vi "Scan with scanning mirror_center point_ver4.0.vi"(8 "Y Scan range (V)":dbl=0.2 min=-200.0 max=300.0, 9 "X Scan range (V)":dbl=0.2 min=-200.0 max=300.0, 10 "Y center (V)":dbl min=-200.0 max=300.0, 11 "X center (V)":dbl min=-200.0 max=300.0) -> ()   [LabVIEW 2015]
uses:
  DNV_YTW/SR400/Public/Typedefs/Counter.ctl
  <vilib>/Analysis/1siggen.llb/Ramp Pattern by Samples.vi
  <vilib>/Analysis/NI_AALBase.lvlib
  DNV_YTW/SR400/SR400.lvlib
panel:
  in  "file path":path
  out "SR400 counts":dbl
  in  "STOP\nSCAN":bool
  in  "Position from":enum16{"Left", "Right", "Control"}(ring)
  in  "Scan select":enum16{"Left", "Right"}(ring)
  in  "Position select":enum16{"Left", "Right", "Zero", "Control"}(ring)
  out "Current Y position (V)":dbl format="%#_4g"
  out "Current X position (V)":dbl format="%#_4g"
  out "Cursor_Y (V) 2":dbl format="%#.5f"
  out "Cursor_X (V) 2":dbl format="%#.5f"
  out "Cursor_Y position 2":i32
  out "Cursor_X position 2":i32
  out "X_Array 2":dbl[](array[numeric])
  out "Y_Array 2":dbl[](array[numeric])
  out "Rescanned Intensity Graph":dbl[][](graph)
  out "Count plot":dbl(graph)=137.0
  in  "stop monitoring":bool
  in  "Log":bool
  out "X_Array":dbl[](array[numeric])
  out "Y_Array":dbl[](array[numeric])
  in  "Scan":bool
  out "Cursor_Y (V)":dbl format="%#.5f"
  out "Cursor_X (V)":dbl format="%#.5f"
  in  "Go":bool
  in  "Stop program":bool
  out "Cursor_Y position":i32
  out "Cursor_X position":i32
  in  "Count Time Set":dbl[unit]=0.01
  in  "# of average":i32=1
  in  "VISA resource name":refnum<visa-resource-name>="GPIB0::23::INSTR"
  out "Counts":dbl
  in  "Time delay bet. movement\n& measurement (ms)":i32=1
  in  "X data number(Ao1)":i32=150
  out "Max Value":dbl format="%#.2p"
  out "Max Y (V)":dbl format="%#.5f"
  out "Max X (V)":dbl format="%#.5f"
  out "Intensity Graph":dbl[][](graph)
  out "ao1_V":dbl
  out "ao1_index":i32
  out "ao0_V":dbl
  out "ao0_index":i32
  in  "Y data number(Ao0)":i32=150
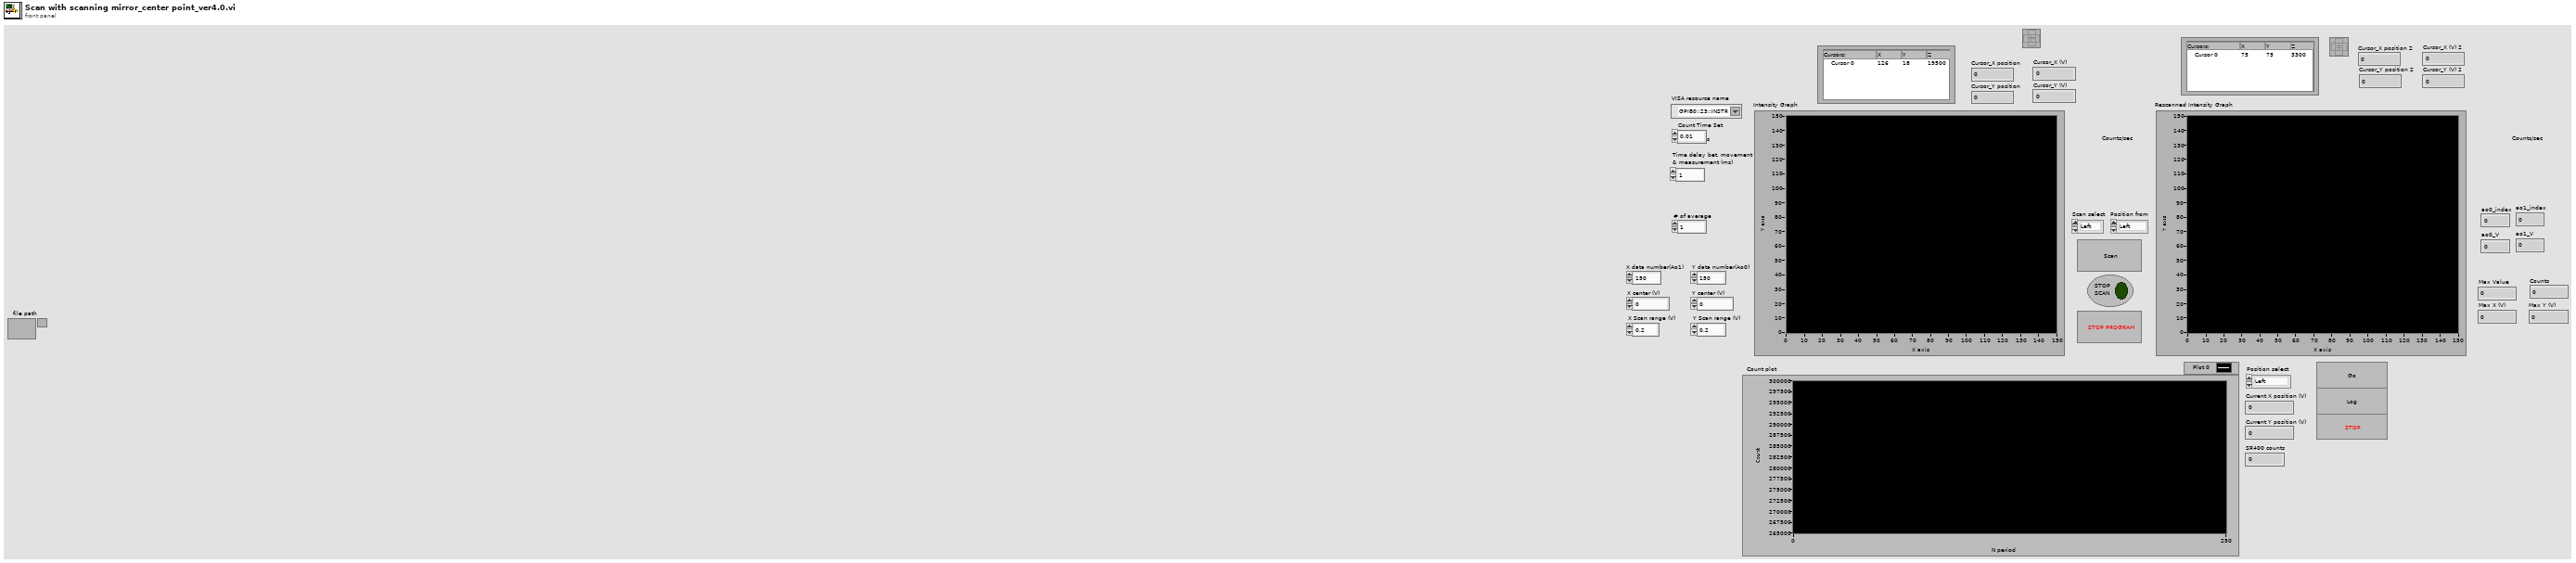
[diagram p1: front panel]
types:
  T1 = enum16{"open", "open or create", "create or replace", "create", "open (read only)"}
  T2 = typedef "SR400.lvlib/Counter.ctl" = enum16{"Counter A", "Counter B", "Counter T"}
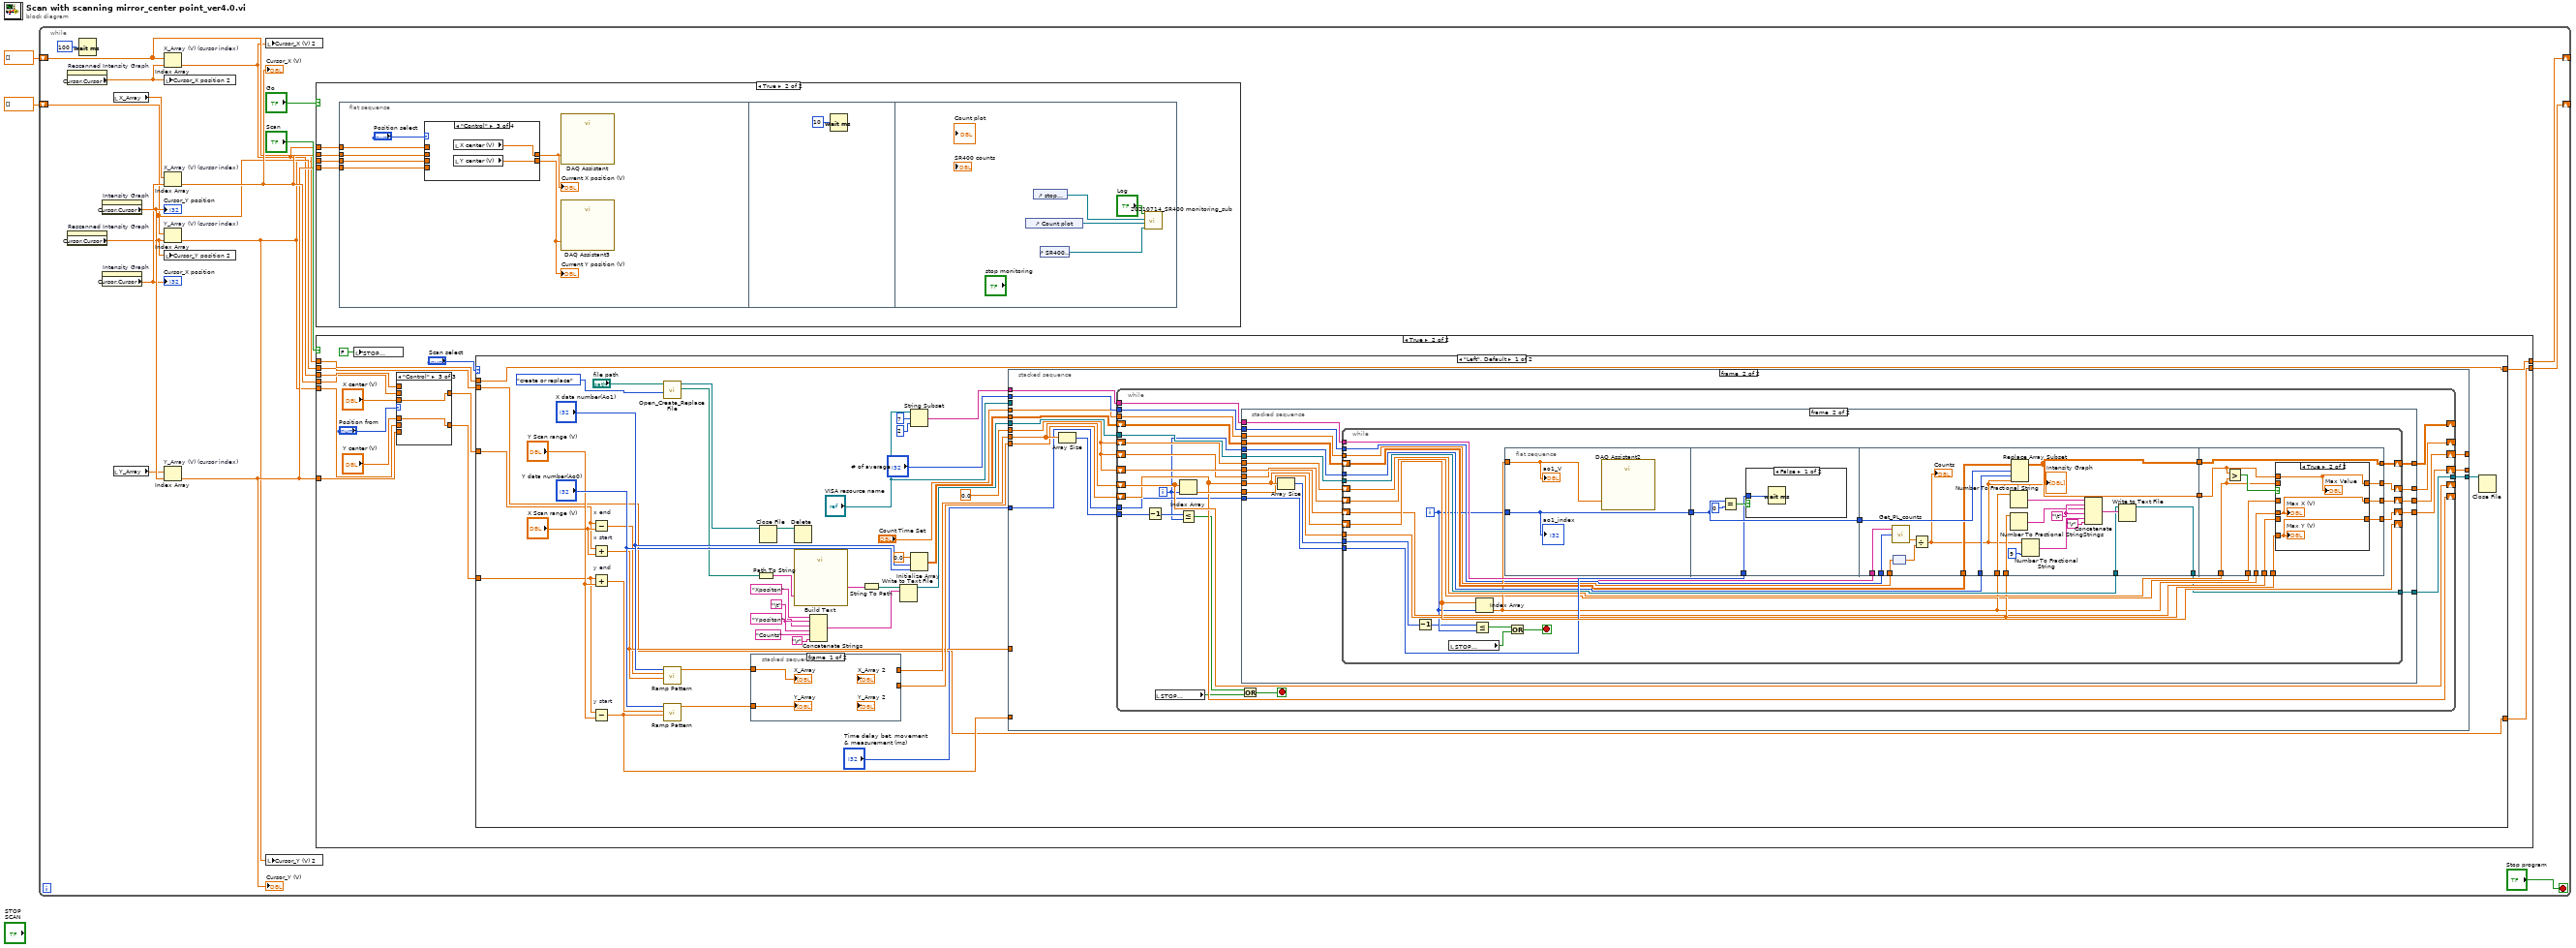
[diagram p0: block diagram]
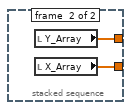
[diagram p5: hidden frame]
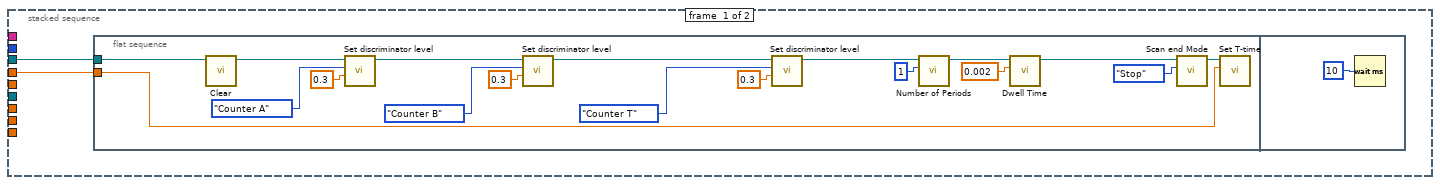
[diagram p6: hidden frame]
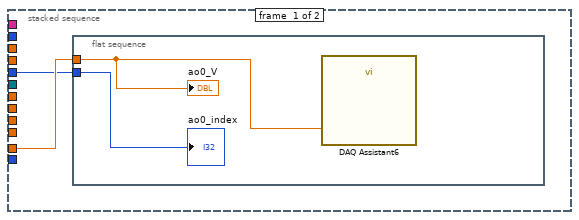
[diagram p7: hidden frame]
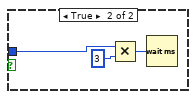
[diagram p8: hidden frame]
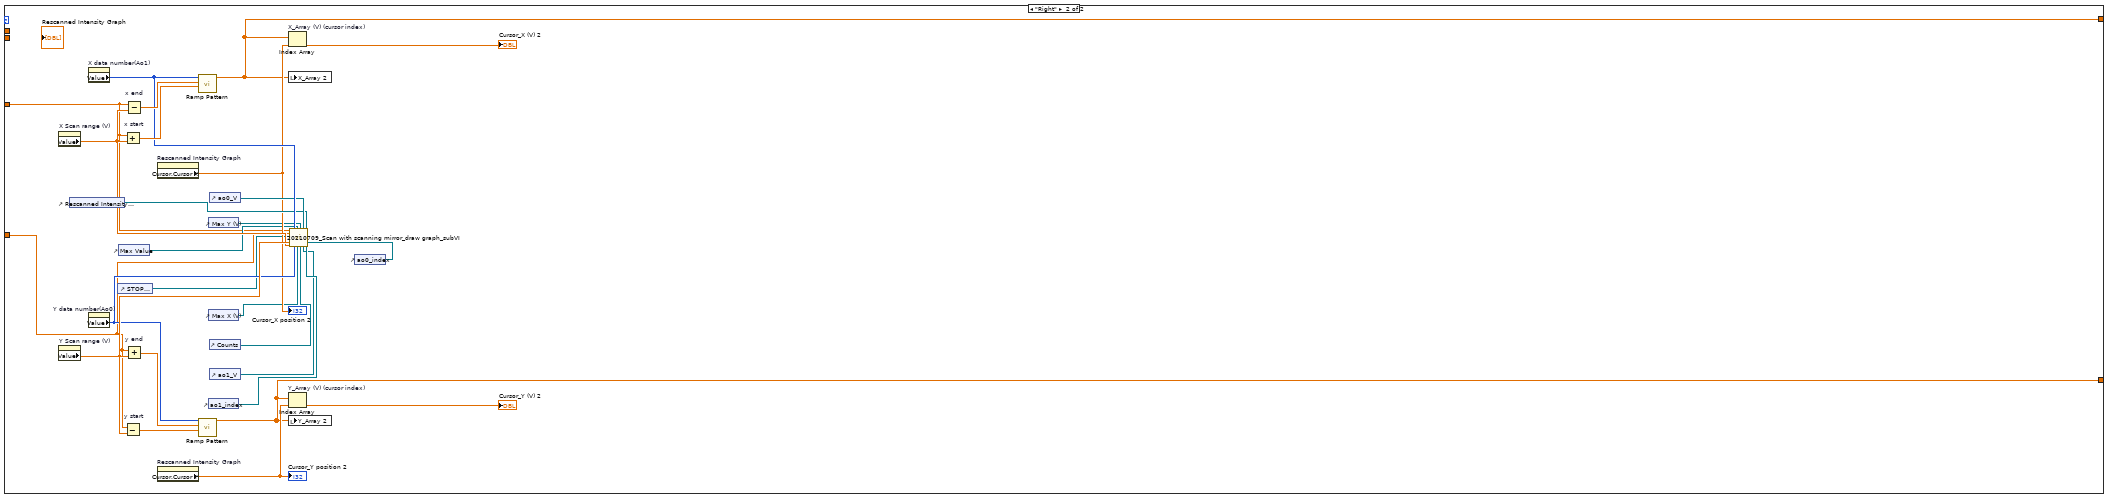
[diagram p10: hidden frame]
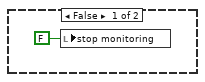
[diagram p11: hidden frame]
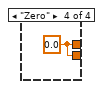
[diagram p14: hidden frame]
diagram:
  n1 = while {
    shift-right: [w10] -> _
    shift-left: dbl[] [] ("Ramp Pattern") -> [w6]
    shift-right: [w7] -> _
    shift-left: dbl[] [] ("Ramp Pattern") -> [w5]
    stop <- "Stop program" stop-if-true
    n2 = property on="Rescanned Intensity Graph" class="IntGraph (strict)"() -> ("Cursor.Cursor X"=w9:dbl)  [unwired: 2 in, 2 out]
    n3 = property on="Rescanned Intensity Graph" class="IntGraph (strict)"() -> ("Cursor.Cursor Y"=w8:dbl)  [unwired: 2 in, 2 out]
    n4 = Wait (ms)(milliseconds to wait=u32 100) -> ()  [unwired: 1 out]
    n5 = property on="Intensity Graph" class="IntGraph (strict)"() -> ("Cursor.Cursor Y"=w17:dbl)  [unwired: 2 in, 2 out]
    "Cursor_Y position" <- w17
    n6 = property on="Intensity Graph" class="IntGraph (strict)"() -> ("Cursor.Cursor X"=w16:dbl)  [unwired: 2 in, 2 out]
    "Cursor_X position" <- w16
    n7 = local read "X_Array"() -> (w15:dbl[])
    n8 = local read "Y_Array"() -> (w14:dbl[])
    n9 = Index Array "X_Array (V) (cursor index)"(array=w6, index=w9) -> (element=w4:dbl)
    n10 = local write "Cursor_X position 2"(w9) -> ()
    n11 = Index Array "X_Array (V) (cursor index)"(array=w15, index=w16) -> (element=w12:dbl)
    "Cursor_X (V)" <- w12
    n12 = Index Array "Y_Array (V) (cursor index)"(array=w5, index=w8) -> (element=w3:dbl)
    n13 = local write "Cursor_Y position 2"(w8) -> ()
    n14 = Index Array "Y_Array (V) (cursor index)"(array=w14, index=w17) -> (element=w11:dbl)
    "Cursor_Y (V)" <- w11
    n15 = local write "Cursor_X (V) 2"(w4) -> ()
    n16 = local write "Cursor_Y (V) 2"(w3) -> ()
    n17 = case shown="True" "Go" {
      tunnel: w12 -> [_ w275]
      tunnel: w11 -> [_ w274]
      tunnel: w4 -> [_ w273]
      tunnel: w3 -> [_ w272]
      frame False {
        n18 = local write "stop monitoring"(FALSE ("monitoring stop")) -> ()
      }
      frame True {
        n19 = flat-sequence {
          tunnel: w275 -> [w281]
          tunnel: w274 -> [w280]
          tunnel: w273 -> [w279]
          tunnel: w272 -> [w278]
          frame #0 {
            n20 = case shown="\"Control\"" "Position select" {
              tunnel: w281 -> [w284 _ _ _]
              tunnel: w280 -> [w283 _ _ _]
              tunnel: w279 -> [_ w286 _ _]
              tunnel: w278 -> [_ w285 _ _]
              tunnel: [w284 w286 w287 w289] -> w277
              tunnel: [w283 w285 w288 w289] -> w276
              frame "Left", Default {
              }
              frame "Right" {
              }
              frame "Control" {
                n21 = local read "X center (V)"() -> (w287:dbl)
                n22 = local read "Y center (V)"() -> (w288:dbl)
              }
              frame "Zero" {
                w289 = 0.0
              }
            }
            "Current X position (V)" <- w277
            "Current Y position (V)" <- w276
            n23 = call "DAQ Assistant"("data"=w277) -> ()  [unwired: 17 in, 2 out]
            n24 = call "DAQ Assistant3"("data"=w276) -> ()  [unwired: 17 in, 2 out]
          }
          frame #1 {
            n25 = Wait (ms)(milliseconds to wait=u32 10) -> ()  [unwired: 1 out]
          }
          frame #2 {
            n26 = control-ref of="Count plot"() -> (w294:refnum<vi>)
            n27 = control-ref of="stop monitoring"() -> (w293:refnum<vi>)
            n28 = control-ref of="SR400 counts"() -> (w291:refnum<vi>)
            n29 = call "20210714_SR400 monitoring_sub.vi"("DigNum Refnum"=w291, "Ctl Refnum"=w294, "stop Refnum"=w293, 11:"Log") -> ()  [unwired: 8 in]
          }
        }
      }
    }
    n30 = case shown="True" "Scan" {
      tunnel: w11 -> [_ w28]
      tunnel: w12 -> [_ w30]
      tunnel: [w22 w37] -> w10
      tunnel: [w21 w36] -> w7
      tunnel: w6 -> [w22 w34]
      tunnel: w5 -> [w21 w33]
      tunnel: w4 -> [_ w31]
      tunnel: w3 -> [_ w29]
      frame False {
      }
      frame True {
        n31 = local write "STOP\nSCAN"(FALSE ("STOP SCAN")) -> ()
        n32 = case shown="\"Control\"" "Position from" {
          tunnel: [w39 w41 w43] -> w27
          tunnel: w30 -> [w39 _ _]
          tunnel: w28 -> [w38 _ _]
          tunnel: [w38 w40 w42] -> w26
          tunnel: w31 -> [_ w41 _]
          tunnel: w29 -> [_ w40 _]
          tunnel: "X center (V)" -> [_ _ w43]
          tunnel: "Y center (V)" -> [_ _ w42]
          frame "Left", Default {
          }
          frame "Right" {
          }
          frame "Control" {
          }
        }
        n33 = case shown="\"Left\", Default" "Scan select" {
          tunnel: [w59 w251] -> w37
          tunnel: [w58 w250] -> w36
          tunnel: w34 -> [w59 _]
          tunnel: w33 -> [w58 _]
          tunnel: w27 -> [w53 w247]
          tunnel: w26 -> [w52 w246]
          frame "Left", Default {
            w65 = "\t"
            n34 = Subtract "x end"(x=w53, y="X Scan range (V)") -> (x-y=w72:dbl)
            n35 = Add "x start"(x=w53, y="X Scan range (V)") -> (x+y=w73:dbl)
            n36 = Add "y end"(x=w52, y="Y Scan range (V)") -> (x+y=w71:dbl)
            n37 = Subtract "y start"(x=w52, y="Y Scan range (V)") -> (x-y=w70:dbl)
            n38 = call <vilib>:"Open_Create_Replace File.vi"("function (open:0)"=T1."create or replace", "file path"="file path") -> ("new file path"=w50:path, "refnum"=w46:refnum<file>)  [unwired: 6 in, 2 out]
            n39 = call-poly <vilib>:"Ramp Pattern.vi"("start"=w73, "end"=w72, "samples"="X data number(Ao1)") -> ("Ramp Pattern"=w85:dbl[])  [unwired: 7 in, 1 out]
            n40 = call-poly <vilib>:"Ramp Pattern.vi"("start"=w70, "end"=w71, "samples"="Y data number(Ao0)") -> ("Ramp Pattern"=w84:dbl[])  [unwired: 7 in, 1 out]
            n41 = stacked-sequence {
              tunnel: [_ w89] -> w82
              tunnel: [_ w88] -> w83
              tunnel: w84 -> [w87 _]
              tunnel: w85 -> [w86 _]
              frame #0 {
                "Y_Array" <- w87
                "X_Array" <- w86
              }
              frame #1 {
                n42 = local read "Y_Array"() -> (w89:dbl[])
                n43 = local read "X_Array"() -> (w88:dbl[])
              }
            }
            n44 = Path To String(path=w50) -> (string=w45:string)
            n45 = Close File(refnum=w46) -> (path=w47:path)  [unwired: 1 in, 1 out]
            n46 = Delete(path (use dialog)=w47) -> ()  [unwired: 4 in, 3 out]
            n47 = call "Build Text"("a"=w45) -> ("Result"=w51:string)  [unwired: 13 in, 1 out]
            n48 = Concatenate Strings("Xpositon" ("string"), w65, "Ypositon" ("string"), w65, "Counts" ("string"), "\r") -> (w62:string)
            n49 = String To Path(string=w51) -> (path=w44:path)
            n50 = Write to Text File(file (use dialog)=w44, text=w62) -> (refnum out=w68:refnum<file>)  [unwired: 2 in, 2 out]
            n51 = String Subset(string="VISA resource name", offset (0)=7, length (rest)=2 ("length (rest)")) -> (substring=w55:string)
            n52 = Initialize Array(0.0, "X data number(Ao1)", "Y data number(Ao0)") -> (w77:dbl[][])
            n53 = stacked-sequence {
              tunnel: w82 -> [_ w123]
              tunnel: w83 -> [_ w122]
              tunnel: "Time delay bet. movement\n& measurement (ms)" -> [_ w121]
              tunnel: w55 -> [_ w120]
              tunnel: w77 -> [_ w119]
              tunnel: w68 -> [_ w118]
              tunnel: [_ w117] -> w69
              tunnel: w73 -> [_ _]
              tunnel: w70 -> [_ _]
              tunnel: 0.0 -> [_ w116]
              tunnel: [_ w115] -> _
              tunnel: [_ w114] -> _
              tunnel: "# of average" -> [_ w113]
              tunnel: "Count Time Set" -> [w91 w111]
              tunnel: "VISA resource name" -> [w90 _]
              frame #0 {
                n54 = flat-sequence {
                  tunnel: w91 -> [w93]
                  tunnel: w90 -> [w92]
                  frame #0 {
                    n55 = call "Clear.vi"("VISA resource name"=w92) -> ("VISA resource name out"=w109:refnum<visa-resource-name>)  [unwired: 9 in, 1 out]
                    n56 = call "Set discriminator level.vi"("Level (-0.034 V)"=0.3, "Discriminator (def: A)"=Counter."Counter A", "VISA resource name"=w109) -> ("VISA resource name out"=w106:refnum<visa-resource-name>)  [unwired: 7 in, 1 out]
                    n57 = call "Set discriminator level.vi"("Level (-0.034 V)"=0.3, "Discriminator (def: A)"=Counter."Counter B", "VISA resource name"=w106) -> ("VISA resource name out"=w103:refnum<visa-resource-name>)  [unwired: 7 in, 1 out]
                    n58 = call "Set discriminator level.vi"("Level (-0.034 V)"=0.3, "Discriminator (def: A)"=Counter."Counter T", "VISA resource name"=w103) -> ("VISA resource name out"=w100:refnum<visa-resource-name>)  [unwired: 7 in, 1 out]
                    n59 = call "Number of Periods.vi"("# of periods (def: 1)"=1, "VISA resource name"=w100) -> ("VISA resource name out"=w98:refnum<visa-resource-name>)  [unwired: 8 in, 1 out]
                    n60 = call "Dwell Time.vi"("Dwell time (0.002 s)"=0.002, "VISA resource name"=w98) -> ("VISA resource name out"=w96:refnum<visa-resource-name>)  [unwired: 8 in, 1 out]
                    n61 = call "Scan end Mode.vi"("Scan End Mode (Def: Stop)"=enum16{"Stop", "Start"}."Stop", "VISA resource name"=w96) -> ("VISA resource name out"=w94:refnum<visa-resource-name>)  [unwired: 8 in, 1 out]
                    n62 = call "Set T-time.vi"("Count Time Set"=w93, "VISA resource name"=w94) -> ()  [unwired: 5 in, 3 out]
                  }
                  frame #1 {
                    n63 = Wait (ms)(milliseconds to wait=u32 10) -> ()  [unwired: 1 out]
                  }
                }
              }
              frame #1 {
                n64 = Array Size(array=w123) -> (size(s)=w112:i32)
                n65 = while {
                  shift-right: [w145] -> _
                  shift-left: w123 -> [w145]
                  shift-right: [w144] -> _
                  shift-left: w122 -> [w144]
                  tunnel: w121 -> [w143]
                  tunnel: w120 -> [w142]
                  shift-right: [w139] -> _
                  shift-left: w119 -> [w141]
                  tunnel: w118 -> [w140]
                  tunnel: [w138] -> w117
                  shift-right: [w137] -> w114
                  shift-left: w116 -> [w132]
                  shift-right: [w135] -> _
                  shift-left: w116 -> [w133]
                  shift-right: [w136] -> w115
                  shift-left: w116 -> [w134]
                  tunnel: w113 -> [w131]
                  tunnel: w112 -> [w127]
                  tunnel: w111 -> [w124]
                  i -> [w126]
                  stop <- w125 stop-if-true
                  n66 = Decrement(x=w127) -> (x-1=w128:i32)
                  n67 = local read "STOP\nSCAN"() -> (w130:bool)
                  n68 = Index Array(array=w145, index=w126) -> (element=w146:dbl)
                  n69 = Less Or Equal?(x=w128, y=w126) -> (x <= y?=w129:bool)
                  n70 = stacked-sequence {
                    tunnel: w146 -> [w148 w163]
                    tunnel: w144 -> [_ w168]
                    tunnel: w143 -> [_ w167]
                    tunnel: w126 -> [w147 w165]
                    tunnel: w142 -> [_ w166]
                    tunnel: w141 -> [_ w164]
                    tunnel: w140 -> [_ w162]
                    tunnel: [_ w161] -> w139
                    tunnel: [_ w160] -> w138
                    tunnel: [_ w159] -> w137
                    tunnel: [_ w158] -> w136
                    tunnel: [_ w157] -> w135
                    tunnel: w134 -> [_ w156]
                    tunnel: w133 -> [_ w155]
                    tunnel: w132 -> [_ w154]
                    tunnel: w131 -> [_ w153]
                    tunnel: w124 -> [_ w151]
                    frame #0 {
                      n71 = flat-sequence {
                        tunnel: w148 -> [w149]
                        tunnel: w147 -> [w150]
                        frame #0 {
                          n72 = call "DAQ Assistant6"("data"=w149) -> ()  [unwired: 17 in, 2 out]
                          "ao0_V" <- w149
                          "ao0_index" <- w150
                        }
                      }
                    }
                    frame #1 {
                      n73 = Array Size(array=w168) -> (size(s)=w152:i32)
                      n74 = while {
                        shift-right: [w196] -> _
                        shift-left: w168 -> [w196]
                        tunnel: w167 -> [w195]
                        tunnel: w166 -> [w194]
                        tunnel: w165 -> [w192]
                        shift-right: [w190] -> w161
                        shift-left: w164 -> [w191]
                        tunnel: w163 -> [w184]
                        tunnel: w162 -> [w189]
                        shift-right: [w186] -> w157
                        shift-left: w155 -> [w185]
                        shift-right: [w182] -> w159
                        shift-left: w154 -> [w180]
                        shift-right: [w181] -> w158
                        shift-left: w156 -> [w179]
                        tunnel: [w178] -> w160
                        tunnel: w153 -> [w176]
                        tunnel: w152 -> [w173]
                        tunnel: w151 -> [w169]
                        i -> [w175]
                        stop <- w170 stop-if-true
                        n75 = Decrement(x=w173) -> (x-1=w174:i32)
                        n76 = local read "STOP\nSCAN"() -> (w171:bool)
                        n77 = Less Or Equal?(x=w174, y=w175) -> (x <= y?=w172:bool)
                        n78 = Index Array(array=w196, index=w175) -> (element=w183:dbl)
                        n79 = flat-sequence {
                          tunnel: w183 -> [w198]
                          tunnel: w175 -> [w197]
                          tunnel: [w197] -> w177
                          tunnel: w195 -> [w199]
                          tunnel: [w201] -> w193
                          tunnel: w177 -> [w201]
                          tunnel: w194 -> [w212]
                          tunnel: w193 -> [w227]
                          tunnel: w192 -> [w226]
                          tunnel: w191 -> [w225]
                          tunnel: w183 -> [w217]
                          tunnel: w184 -> [w216]
                          tunnel: w189 -> [w214]
                          tunnel: [w224] -> w188
                          tunnel: [w210] -> w187
                          tunnel: [w213] -> w178
                          tunnel: w176 -> [w211]
                          tunnel: w169 -> [w207]
                          tunnel: [w238] -> w190
                          tunnel: w188 -> [w238]
                          tunnel: w187 -> [w228]
                          tunnel: [w236] -> w186
                          tunnel: w185 -> [w229]
                          tunnel: w184 -> [w235]
                          tunnel: w183 -> [w234]
                          tunnel: [w233] -> w182
                          tunnel: [w232] -> w181
                          tunnel: w180 -> [w231]
                          tunnel: w179 -> [w230]
                          frame #0 {
                            n80 = call "DAQ Assistant2"("data"=w198) -> ()  [unwired: 17 in, 2 out]
                            "ao1_V" <- w198
                            "ao1_index" <- w197
                          }
                          frame #1 {
                            n81 = Equal?(x=w201, y=0) -> (x = y?=w202:bool)
                            n82 = case shown="False" w202 {
                              tunnel: w199 -> [w203 w205]
                              frame False {
                                n83 = Wait (ms)(milliseconds to wait=w203) -> ()  [unwired: 1 out]
                              }
                              frame True {
                                n84 = Multiply(x=w205, y=3) -> (x*y=w206:i32)
                                n85 = Wait (ms)(milliseconds to wait=w206) -> ()  [unwired: 1 out]
                              }
                            }
                          }
                          frame #2 {
                            w223 = "\t"
                            n86 = call "Get_PL_counts.vi"("# of average"=w211, "SR400 GPIB Address"=w212) -> ("Averaged counts"=w209:dbl)  [unwired: 2 in]
                            n87 = node(w207) -> (w208:dbl)
                            n88 = Divide(x=w209, y=w208) -> (x/y=w210:dbl)
                            "Counts" <- w210
                            n89 = Number To Fractional String(number=w217) -> (F-format string=w218:string)  [unwired: 3 in]
                            n90 = Number To Fractional String(number=w216) -> (F-format string=w215:string)  [unwired: 3 in]
                            n91 = Replace Array Subset(array=w225, new element=w210, index (row)=w227, index (col)=w226) -> (w224:dbl[][])
                            "Intensity Graph" <- w224
                            n92 = Number To Fractional String(number=w210, precision (6)=i16 9) -> (F-format string=w219:string)  [unwired: 2 in]
                            n93 = Concatenate Strings(w218, w223, w215, w223, w219, "\r") -> (w221:string)
                            n94 = Write to Text File(file (use dialog)=w214, text=w221) -> (refnum out=w213:refnum<file>)  [unwired: 2 in, 2 out]
                          }
                          frame #3 {
                            n95 = Greater?(x=w228, y=w229) -> (0:w237:bool)
                            n96 = case shown="True" w237 {
                              tunnel: w228 -> [_ w244]
                              tunnel: [w241 w244] -> w236
                              tunnel: w229 -> [w241 _]
                              tunnel: w235 -> [_ w243]
                              tunnel: w234 -> [_ w242]
                              tunnel: [w240 w243] -> w233
                              tunnel: [w239 w242] -> w232
                              tunnel: w231 -> [w240 _]
                              tunnel: w230 -> [w239 _]
                              frame False {
                              }
                              frame True {
                                "Max Value" <- w244
                                "Max Y (V)" <- w243
                                "Max X (V)" <- w242
                              }
                            }
                          }
                        }
                        n97 = Or(x=w172, y=w171) -> (x .or. y?=w170:bool)
                      }
                    }
                  }
                  n98 = Or(x=w129, y=w130) -> (x .or. y?=w125:bool)
                }
              }
            }
            n99 = Close File(refnum=w69) -> ()  [unwired: 1 in, 2 out]
          }
          frame "Right" {
            n100 = property on="X Scan range (V)" class="DigNum (strict)"() -> ("Value"=w266:dbl)  [unwired: 2 in, 2 out]
            n101 = property on="Y Scan range (V)" class="DigNum (strict)"() -> ("Value"=w270:dbl)  [unwired: 2 in, 2 out]
            n102 = control-ref of="Rescanned Intensity Graph"() -> (w258:refnum<vi>)
            n103 = property on="X data number(Ao1)" class="DigNum (strict)"() -> ("Value"=w263:i32)  [unwired: 2 in, 2 out]
            n104 = property on="Y data number(Ao0)" class="DigNum (strict)"() -> ("Value"=w267:i32)  [unwired: 2 in, 2 out]
            n105 = control-ref of="STOP\nSCAN"() -> (w245:refnum<vi>)
            n106 = control-ref of="Max Value"() -> (w249:refnum<vi>)
            n107 = Add "x start"(x=w247, y=w266) -> (x+y=w264:dbl)
            n108 = Subtract "y start"(x=w246, y=w270) -> (x-y=w268:dbl)
            n109 = Subtract "x end"(x=w247, y=w266) -> (x-y=w265:dbl)
            n110 = Add "y end"(x=w246, y=w270) -> (x+y=w269:dbl)
            n111 = property on="Rescanned Intensity Graph" class="IntGraph (strict)"() -> ("Cursor.Cursor X"=w257:dbl)  [unwired: 2 in, 2 out]
            "Cursor_X position 2" <- w257
            n112 = property on="Rescanned Intensity Graph" class="IntGraph (strict)"() -> ("Cursor.Cursor Y"=w256:dbl)  [unwired: 2 in, 2 out]
            "Cursor_Y position 2" <- w256
            n113 = call-poly <vilib>:"Ramp Pattern.vi"("start"=w264, "end"=w265, "samples"=w263) -> ("Ramp Pattern"=w251:dbl[])  [unwired: 7 in, 1 out]
            n114 = call-poly <vilib>:"Ramp Pattern.vi"("start"=w268, "end"=w269, "samples"=w267) -> ("Ramp Pattern"=w250:dbl[])  [unwired: 7 in, 1 out]
            n115 = control-ref of="Max Y (V)"() -> (w252:refnum<vi>)
            n116 = control-ref of="Max X (V)"() -> (w253:refnum<vi>)
            n117 = control-ref of="ao1_index"() -> (w262:refnum<vi>)
            n118 = control-ref of="ao0_V"() -> (w260:refnum<vi>)
            n119 = control-ref of="Counts"() -> (w248:refnum<vi>)
            n120 = control-ref of="ao1_V"() -> (w259:refnum<vi>)
            n121 = Index Array "X_Array (V) (cursor index)"(array=w251, index=w257) -> (element=→"Cursor_X (V) 2":dbl)
            n122 = local write "X_Array 2"(w251) -> ()
            n123 = Index Array "Y_Array (V) (cursor index)"(array=w250, index=w256) -> (element=→"Cursor_Y (V) 2":dbl)
            n124 = local write "Y_Array 2"(w250) -> ()
            n125 = control-ref of="ao0_index"() -> (w261:refnum<vi>)
            n126 = call "20210709_Scan with scanning mirror_draw graph_subVI.vi"("X center (V)"=w247, "Y center (V)"=w246, "Bool Refnum"=w245, "X Scan range (V)"=w270, "Y Scan range (V)"=w266, "X data number(Ao1)"=w263, "Y data number(Ao0)"=w267, "DigNum Refnum 7"=w249, "DigNum Refnum 4"=w253, "DigNum Refnum 3"=w252, "DigNum Refnum 8"=w248, "DigNum Refnum 5"=w260, "DigNum Refnum 6"=w259, "IntGraph Refnum"=w258, "DigNum Refnum"=w261, "DigNum Refnum 2"=w262) -> ()  [unwired: 3 in, 1 out]
          }
        }
      }
    }
  }
